vi "Interface.vi"(9 "EventsIn":T1, 10 "Events":T2) -> ()   [LabVIEW 2015, in "TemplatePlugin.lvlib" / "TemplatePlugin.lvclass"]
uses:
  TemplatePlugin.lvclass
  <resource>/Framework/Providers/Veritech_GCM/Support/Framework/_Plugins/_LVCMPlugin/GCMPlugin_EventsOut.ctl
  <resource>/Framework/Providers/Veritech_GCM/Support/Framework/_Plugins/_LVCMPlugin/GCMPlugin_EventsIn.ctl
  <resource>/Framework/Providers/Veritech_GCM/Support/Framework/_Plugins/GCMPlugin/GCMPlugin.lvclass
types:
  T1 = typedef "GCMPlugin.lvclass/GCMPlugin_EventsIn.ctl" = cluster{"Stop":refnum<user-event>, "ItemSelected":refnum<user-event>, "ItemDeselected":refnum<user-event>, "PluginActivated":refnum<user-event>, "PluginDeactivated":refnum<user-event>}
  T2 = typedef "GCMPlugin.lvclass/GCMPlugin_EventsOut.ctl" = cluster{"ItemEdited":refnum<user-event>}
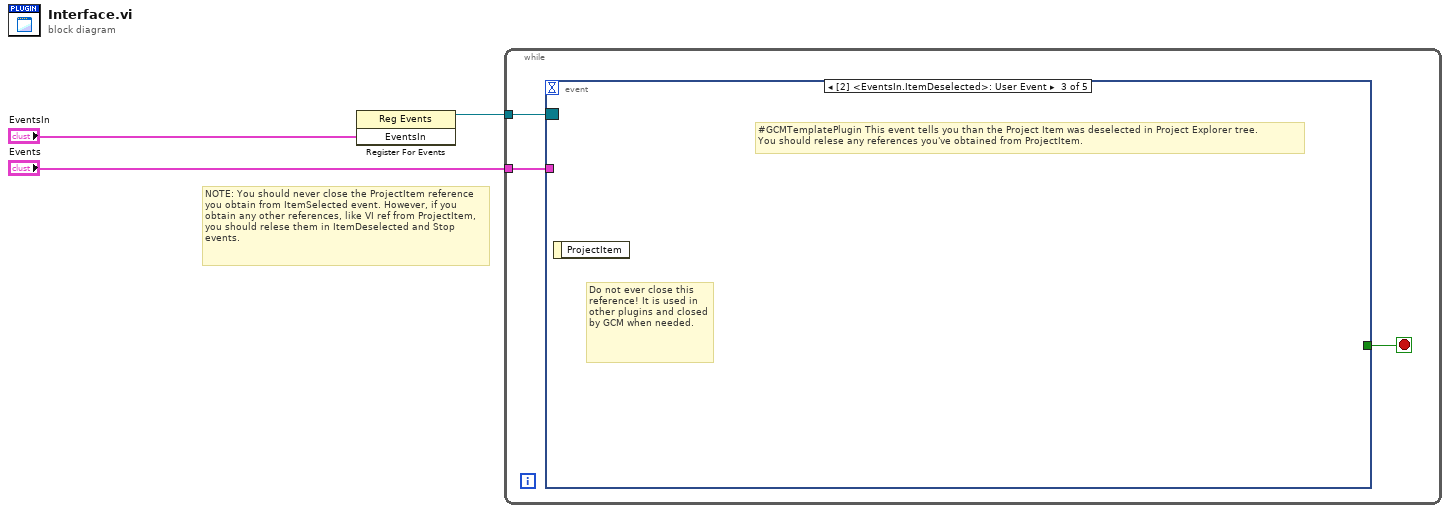
[diagram p0: block diagram]
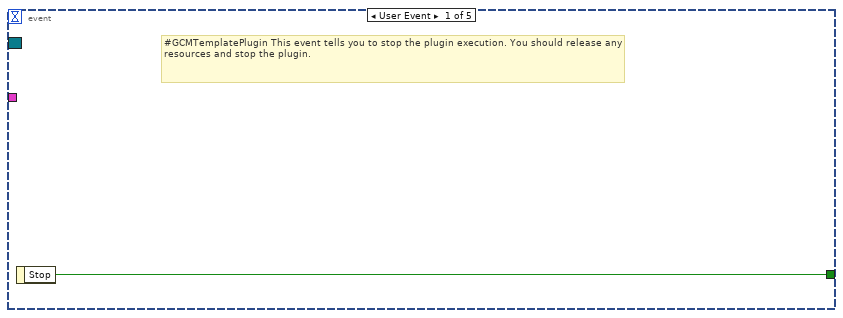
[diagram p2: hidden frame]
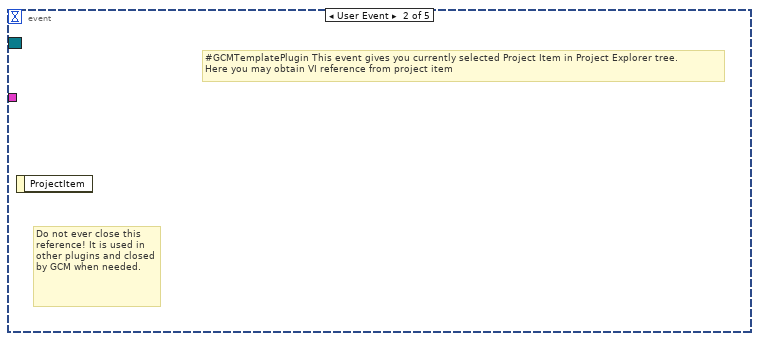
[diagram p3: hidden frame]
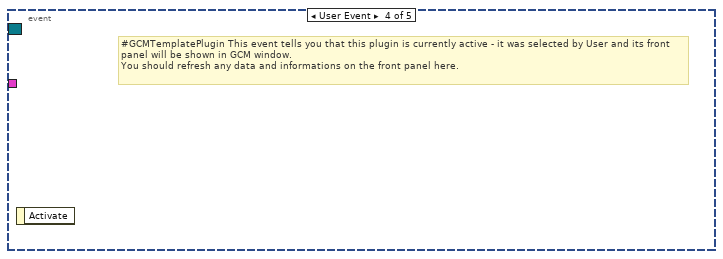
[diagram p4: hidden frame]
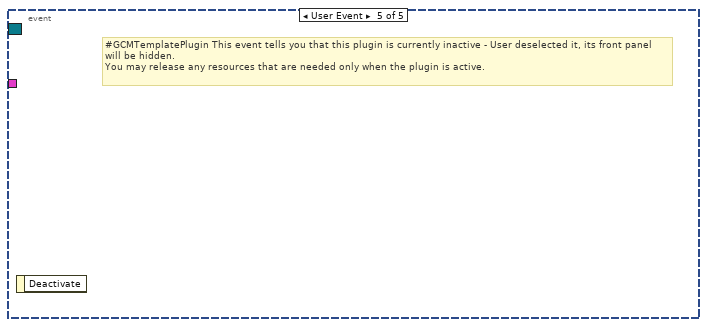
[diagram p5: hidden frame]
diagram:
  # "NOTE: You should never close the ProjectItem reference you obtain from ItemSelected event. However, if you obtain any other references, like VI ref from ProjectItem, you should relese them in ItemDeselected and Stop events."
  n1 = register-events("EventsIn") -> (reference out=w2:refnum<event-registration>)  [unwired: 2 in, 1 out]
  n2 = while {
    tunnel: w2 -> [w6]
    tunnel: "Events" -> [w5]
    stop <- w4 stop-if-true
    n3 = event shown="[2] <EventsIn.ItemDeselected>: User Event" {
      selector: w6 -> [_ _ _ _ _]
      dyn-events: _ -> [_ _ _ _ _]
      timeout: _ -> [_ _ _ _ _]
      tunnel: w5 -> [_ _ _ _ _]
      tunnel: [w7 _ _ _ _] -> w4
      event User Event {
        # "#GCMTemplatePlugin This event tells you to stop the plugin execution. You should release any resources and stop the plugin."
        n4 = event-data() -> ("Stop"=w7:bool)  [unwired: 1 in]
      }
      event User Event {
        # "Do not ever close this reference! It is used in other plugins and closed by GCM when needed."
        # "#GCMTemplatePlugin This event gives you currently selected Project Item in Project Explorer tree.\nHere you may obtain VI reference from project item"
        n5 = event-data() -> ()  [unwired: 1 in, 1 out]
      }
      event User Event {
        # "Do not ever close this reference! It is used in other plugins and closed by GCM when needed."
        # "#GCMTemplatePlugin This event tells you than the Project Item was deselected in Project Explorer tree.\nYou should relese any references you've obtained from ProjectItem."
        n6 = event-data() -> ()  [unwired: 1 in, 1 out]
      }
      event User Event {
        # "#GCMTemplatePlugin This event tells you that this plugin is currently active - it was selected by User and its front panel will be shown in GCM window.\nYou should refresh any data and informations on the front panel here."
        n7 = event-data() -> ()  [unwired: 1 in, 1 out]
      }
      event User Event {
        # "#GCMTemplatePlugin This event tells you that this plugin is currently inactive - User deselected it, its front panel will be hidden.\nYou may release any resources that are needed only when the plugin is active."
        n8 = event-data() -> ()  [unwired: 1 in, 1 out]
      }
    }
  }
